vi "Humidity_Testcode.vi"() -> ()   [LabVIEW 2024]
uses:
  <vilib>/Instr/_visa.llb/VISA Find Search Mode.ctl
  98437b02-8359-4557-a993-eca74e982cb1.vi
  <vilib>/Instr/_visa.llb/VISA Configure Serial Port (Instr).vi
  <vilib>/regexp/Match Regular Expression.xnode
panel:
  in  "stop":bool
  out "RH":dbl
  out "RH[%]":string
  out "AT":dbl
  out "AT[C]":string
  out "DP":dbl
  out "DP[C]":string
  out "Redo the task":string="Humidity: Connect"
  out "find list":string[](array[string])
  out "Serial Settings:Number of Bytes at Serial Port":u32
  out "VISA resource name":refnum<visa-resource-name>
  out "Connection":bool
  out "Receved":bool
  out "error out":errorcluster
  out "Serial Settings:Baud Rate":u32
  out "read buffer":string
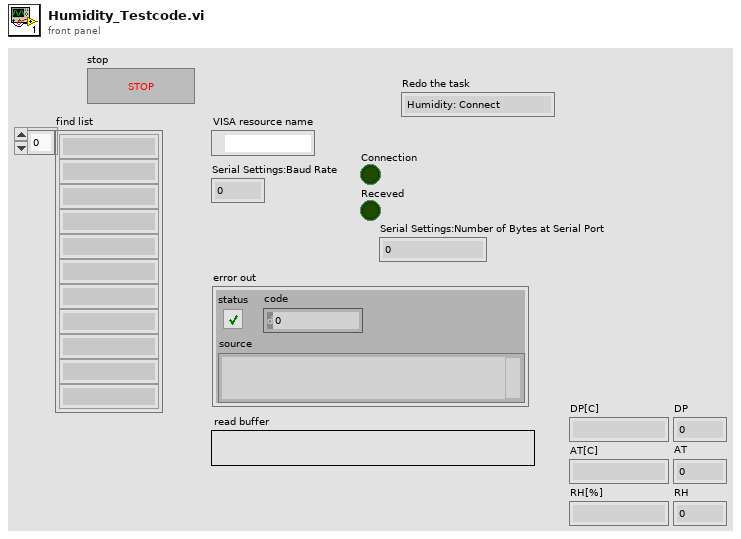
[diagram p1: front panel]
types:
  T1 = typedef "VISA Find Search Mode.ctl" = u32
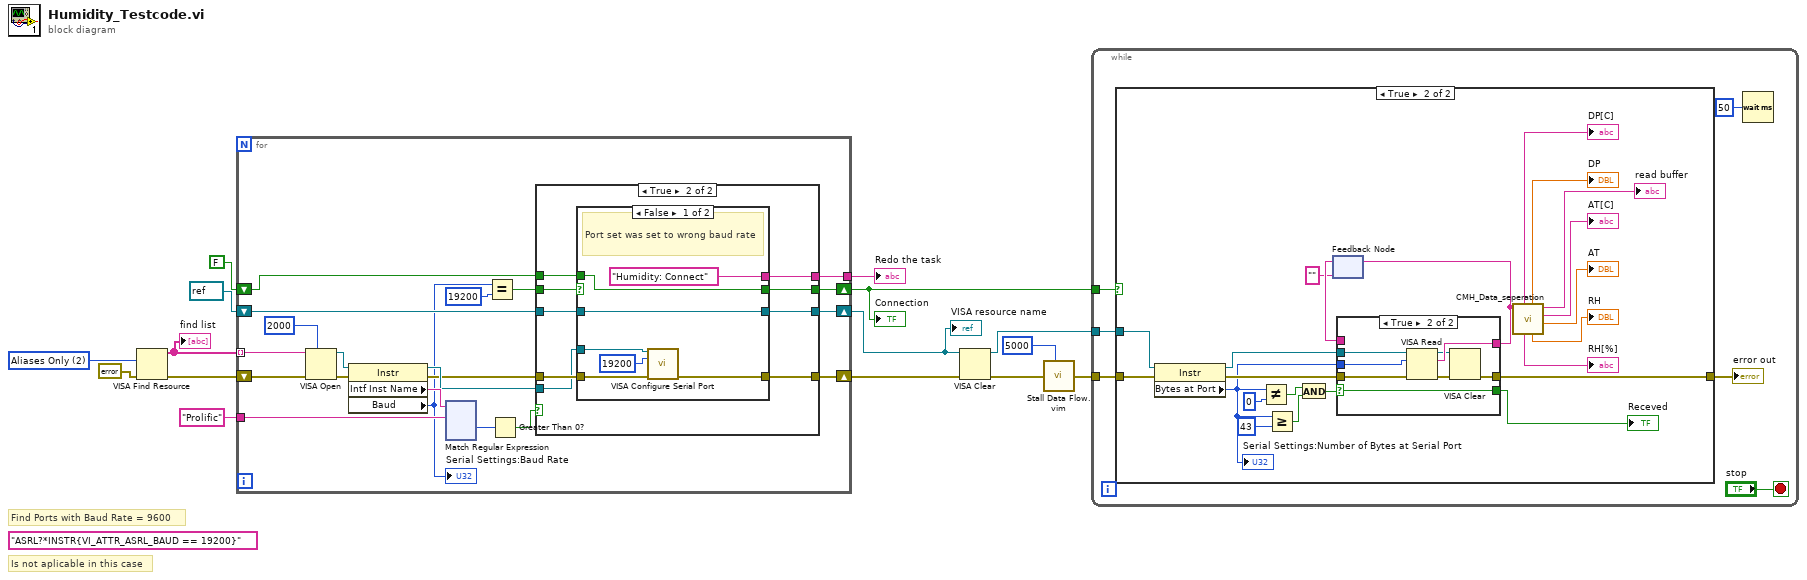
[diagram p0: block diagram]
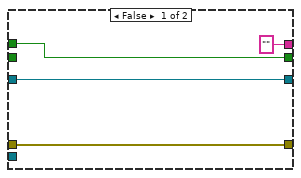
[diagram p4: hidden frame]
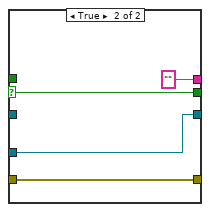
[diagram p5: hidden frame]
diagram:
  (unwired) "ASRL?*INSTR{VI_ATTR_ASRL_BAUD == 19200}" ("expression (\"?*\")")
  w15 = T1 2 items=["Canonical Names Only"=0, "Aliases Only"=2, "Include Matching Aliases"=3, "Include All Aliases"=4] ("Search Mode")
  # "Is not aplicable in this case"
  # "Find Ports with Baud Rate = 9600"
  n1 = VISA Find Resource(8:errorcluster {"status"=FALSE, "code"=0, "source"=""} ("error in (no error)"), 10:w15) -> (0:w11:errorcluster, 3:w10:string[])  [unwired: 1 in, 1 out]
  "find list" <- w10
  n2 = for {
    tunnel: "Prolific" -> [w20]
    shift-right: [w24] -> w6
    shift-left: refnum<visa-resource-name> refnum ("VISA resource name") -> [w23]
    shift-right: [w21] -> w7
    shift-left: w11 -> [w35]
    shift-right: [w26] -> w9
    shift-left: FALSE -> [w25]
    tunnel: w10 -> [w33] mode=indexing
    tunnel: [w19] -> w5
    n3 = VISA Open(timeout (0)=u32 2000 ("VISA Open timeout (0)"), error in (no error)=w35, VISA resource name=w33) -> (VISA resource name=w32:refnum<visa-resource-name>, error out=w29:errorcluster)  [unwired: 2 in]
    n4 = property class="Instr"(reference=w32, error in=w29) -> (reference out=w27:refnum<visa-resource-name>, error out=w22:errorcluster, "Intf Inst Name"=w28:string, "Baud"=w17:u32)
    "Serial Settings:Baud Rate" <- w17
    n5 = xnode "Match Regular Expression"("input string"=w28, "regular expression"=w20) -> ("offset past match"=w31:i32)  [unwired: 4 in, 4 out]
    n6 = Equal?(x=w17, y=u32 19200) -> (x = y?=w16:bool)
    n7 = Greater Than 0?(x=w31) -> (x > 0?=w34:bool)
    n8 = case shown="True" w34 {
      tunnel: w27 -> [_ w47]
      tunnel: [w39 w42] -> w26
      tunnel: w25 -> [w39 w41]
      tunnel: [w38 w46] -> w24
      tunnel: w23 -> [w38 w43]
      tunnel: w22 -> [w37 w48]
      tunnel: [w37 w45] -> w21
      tunnel: w16 -> [_ w44]
      tunnel: ["" w40] -> w19
      frame False {
      }
      frame True {
        n9 = case shown="False" w44 {
          selector: w44 -> [_ w57]
          tunnel: w48 -> [w55 w59]
          tunnel: w47 -> [w54 w58]
          tunnel: [w52 w58] -> w46
          tunnel: [w49 w59] -> w45
          tunnel: w43 -> [w52 _]
          tunnel: [w51 w57] -> w42
          tunnel: w41 -> [w51 _]
          tunnel: ["Humidity: Connect" ""] -> w40
          frame False {
            # "Port set was set to wrong baud rate"
            n10 = call-poly "VISA Configure Serial Port"("VISA resource name"=w54, "baud rate (9600)"=u32 19200, "error in (no error)"=w55) -> ("error out"=w49:errorcluster)  [unwired: 11 in, 1 out]
          }
          frame True {
          }
        }
      }
    }
  }
  "Connection" <- w9
  "VISA resource name" <- w6
  "Redo the task" <- w5
  n11 = VISA Clear(VISA resource name=w6, error in (no error)=w7) -> (VISA resource name out=w4:refnum<visa-resource-name>, error out=w3:errorcluster)
  n12 = call "Stall Data Flow.vim"("value in"=w3, "milliseconds to wait"=u32 5000) -> ("value out"=w1:errorcluster)  [unwired: 1 out]
  n13 = while {
    tunnel: w9 -> [w182]
    tunnel: w4 -> [w180]
    tunnel: w1 -> [w179]
    stop <- "stop" stop-if-true
    n14 = case shown="True" w182 {
      tunnel: [w183 w205] -> w181
      tunnel: w180 -> [_ w191]
      tunnel: w179 -> [w183 w190]
      frame False {
      }
      frame True {
        n15 = property class="Instr"(reference=w191, error in=w190) -> (reference out=w204:refnum<visa-resource-name>, error out=w203:errorcluster, "Bytes at Port"=w189:u32)
        "Serial Settings:Number of Bytes at Serial Port" <- w189
        n16 = Not Equal?(x=w189, y=u32 0) -> (x != y?=w187:bool)
        n17 = Greater Or Equal?(x=w189, y=u32 43) -> (x >= y?=w186:bool)
        n18 = And(x=w187, y=w186) -> (x .and. y?=w185:bool)
        n19 = feedback #1("" ("read buffer")) -> (w193:string)
        n20 = case shown="True" w185 {
          selector: w185 -> [w207 w213]
          tunnel: w204 -> [_ w215]
          tunnel: w203 -> [w208 w216]
          tunnel: [w208 w209] -> w205
          tunnel: w189 -> [_ w214]
          tunnel: [w207 w213] -> w184
          tunnel: [w206 w212] -> w194
          tunnel: w193 -> [w206 _]
          frame False {
          }
          frame True {
            n21 = VISA Read(VISA resource name=w215, byte count=w214, error in (no error)=w216) -> (VISA resource name out=w210:refnum<visa-resource-name>, read buffer=w212:string, error out=w211:errorcluster)  [unwired: 1 out]
            n22 = VISA Clear(VISA resource name=w210, error in (no error)=w211) -> (error out=w209:errorcluster)  [unwired: 1 out]
          }
        }
        "Receved" <- w184
        n23 = feedback-in #1(w194) -> ()
        n24 = call "CMH_Data_seperation.vi"("Humidity readout"=w194) -> ("AT"=→"AT":dbl, "AT[C]"=→"AT[C]":string, "read buffer"=→"read buffer":string, "RH"=→"RH":dbl, "DP"=→"DP":dbl, "RH[%]"=→"RH[%]":string, "DP[C]"=→"DP[C]":string)  [unwired: 3 in, 1 out]
      }
    }
    "error out" <- w181
    n25 = Wait (ms)(milliseconds to wait=u32 50) -> ()  [unwired: 1 out]
  }
